vi "run.vi"(8 "error in (no error)":errorcluster, 11 "Protocol_TwoCreep in":refnum<class "Protocol_TwoCreep.lvclass">) -> (0 "error out":errorcluster, 3 "Protocol_TwoCreep out":refnum<class "Protocol_TwoCreep.lvclass">)   [LabVIEW 2011, in "Protocol_TwoCreep.lvclass"]
uses:
  Protocol_TwoCreep.lvclass
  protocol_Generic/Protocol_Generic.lvclass
  Protocol_TwoCreep.lvclass/Protocol_TwoCreep.ctl
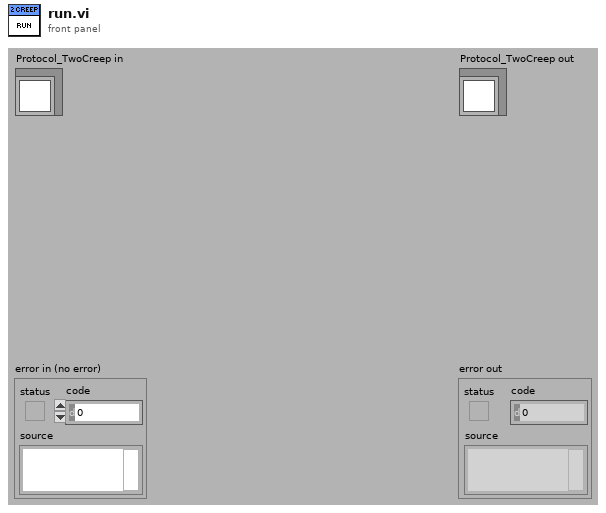
[diagram p1: front panel]
types:
  T1 = cluster{"Set Point":dbl, "Set Point Time":dbl, "Ramp Amplitude":dbl, "Ramp Rate":dbl}
  T2 = cluster{"Axis Information":cluster{"Device ID":i32, "Device Name":string, "Device Type":i32}[], "Axis Selector":i32[], "Control Modes out":u16[], "error out":errorcluster, "Channel Data":cluster{"Name":string, "Type":i32, "SI Full Scale":dbl, "Full Scale":dbl, "Units String":string, "Display Format":string, "Gauge Length":dbl}[][]}
  T3 = cluster{"Device ID":i32, "Device Name":string, "Device Type":i32}[]
  T4 = cluster{"Name":string, "Type":i32, "SI Full Scale":dbl, "Full Scale":dbl, "Units String":string, "Display Format":string, "Gauge Length":dbl}[][]
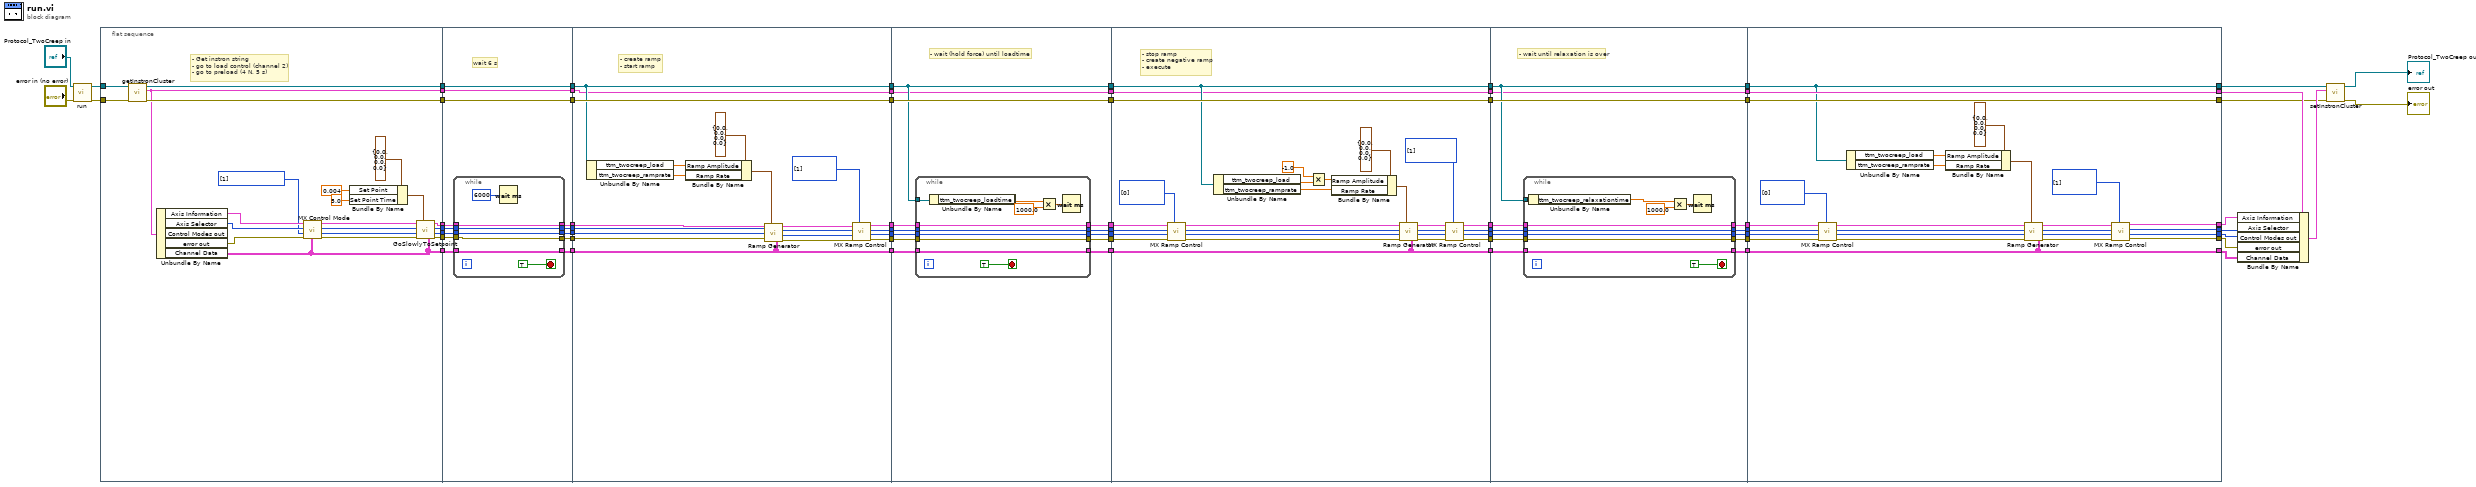
[diagram p0: block diagram]
diagram:
  n1 = call-parent "run.vi"("error in (no error)"="error in (no error)", "Protocol_Generic in"="Protocol_TwoCreep in") -> ("error out"=w60:errorcluster, "Protocol_Generic out"=w61:refnum<class "Protocol_TwoCreep.lvclass">)  [unwired: 8 in]
  n2 = flat-sequence {
    tunnel: w61 -> [w85]
    tunnel: w60 -> [w84]
    tunnel: [w64] -> w59
    tunnel: [w83] -> w58
    tunnel: [w70] -> w57
    tunnel: [w69] -> w56
    tunnel: [w68] -> w55
    tunnel: [w67] -> w54
    tunnel: [w66] -> w47
    tunnel: [w65] -> w17
    tunnel: w59 -> [w98]
    tunnel: w58 -> [w97]
    tunnel: w57 -> [w96]
    tunnel: w56 -> [w95]
    tunnel: w55 -> [w94]
    tunnel: w54 -> [w93]
    tunnel: [w98] -> w53
    tunnel: [w97] -> w52
    tunnel: [w92] -> w51
    tunnel: [w91] -> w50
    tunnel: [w90] -> w49
    tunnel: [w89] -> w48
    tunnel: w47 -> [w88]
    tunnel: [w87] -> w46
    tunnel: w17 -> [w86]
    tunnel: [w86] -> w16
    tunnel: w53 -> [w120]
    tunnel: w52 -> [w126]
    tunnel: w51 -> [w125]
    tunnel: w50 -> [w124]
    tunnel: w49 -> [w123]
    tunnel: w48 -> [w122]
    tunnel: w46 -> [w107]
    tunnel: [w120] -> w45
    tunnel: [w126] -> w44
    tunnel: [w111] -> w43
    tunnel: [w110] -> w42
    tunnel: [w109] -> w41
    tunnel: [w108] -> w40
    tunnel: [w107] -> w39
    tunnel: w16 -> [w106]
    tunnel: [w106] -> w15
    tunnel: w45 -> [w128]
    tunnel: w44 -> [w139]
    tunnel: w43 -> [w133]
    tunnel: w42 -> [w134]
    tunnel: w41 -> [w135]
    tunnel: w40 -> [w136]
    tunnel: w39 -> [w138]
    tunnel: [w128] -> w38
    tunnel: [w139] -> w37
    tunnel: [w137] -> w36
    tunnel: [w132] -> w35
    tunnel: [w131] -> w34
    tunnel: [w130] -> w33
    tunnel: [w129] -> w32
    tunnel: w15 -> [w127]
    tunnel: [w127] -> w13
    tunnel: w38 -> [w163]
    tunnel: w37 -> [w177]
    tunnel: w36 -> [w164]
    tunnel: w35 -> [w176]
    tunnel: w34 -> [w175]
    tunnel: w33 -> [w174]
    tunnel: w32 -> [w173]
    tunnel: [w163] -> w31
    tunnel: [w177] -> w30
    tunnel: [w164] -> w29
    tunnel: [w158] -> w28
    tunnel: [w156] -> w27
    tunnel: [w154] -> w26
    tunnel: [w152] -> w25
    tunnel: [w150] -> w14
    tunnel: w13 -> [w150]
    tunnel: w31 -> [w179]
    tunnel: w30 -> [w190]
    tunnel: w29 -> [w182]
    tunnel: w28 -> [w189]
    tunnel: w27 -> [w187]
    tunnel: w26 -> [w185]
    tunnel: w25 -> [w183]
    tunnel: [w179] -> w24
    tunnel: [w190] -> w23
    tunnel: [w181] -> w22
    tunnel: [w188] -> w21
    tunnel: [w186] -> w20
    tunnel: [w184] -> w19
    tunnel: [w180] -> w18
    tunnel: w14 -> [w178]
    tunnel: [w178] -> w12
    tunnel: [w204] -> w7
    tunnel: [w206] -> w8
    tunnel: [w208] -> w9
    tunnel: [w210] -> w10
    tunnel: [w203] -> w6
    tunnel: [w226] -> w1
    tunnel: [w201] -> w4
    tunnel: w24 -> [w201]
    tunnel: w23 -> [w226]
    tunnel: w22 -> [w203]
    tunnel: w21 -> [w216]
    tunnel: w20 -> [w215]
    tunnel: w19 -> [w214]
    tunnel: w18 -> [w213]
    tunnel: [w202] -> w11
    tunnel: w12 -> [w202]
    frame #0 {
      w79 = u16[] [1] items=["Channel 1", "Channel 2", "Channel 3", "Channel 4"] ("Control Modes")
      # "- Get instron string\n- go to load control (channel 2)\n- go to preload (4 N, 5 s)"
      n3 = call-dynamic "getInstronCluster.vi"("error in (no error)"=w84, "Protocol_Generic in"=w85) -> ("error out"=w83:errorcluster, "InstronCluster"=w65:T2, "Protocol_Generic out"=w64:refnum<class "Protocol_TwoCreep.lvclass">)  [unwired: 7 in]
      n4 = Unbundle By Name(w65) -> ("Axis Information"=w82:T3, "Axis Selector"=w81:i32[], "error out"=w80:errorcluster, "Channel Data"=w66:T4)  [unwired: 1 out]
      n5 = call "MX Control Mode.vi"("Channel Data"=w66, "error in (no error)"=w80, "Control Modes"=w79, "Axis Selector"=w81, "Axis Information"=w82) -> ("error out"=w75:errorcluster, "Control Modes out"=w76:u16[], "Axis Selector out"=w77:i32[], "Axis Information out"=w78:T3)  [unwired: 1 in]
      n6 = Bundle By Name(cluster=T1 {"Set Point"=0.0, "Set Point Time"=0.0, "Ramp Amplitude"=0.0, "Ramp Rate"=0.0} ("Input cluster"), "Set Point"=0.004, "Set Point Time"=5.0) -> (w74:T1)
      n7 = call "GoSlowlyToSetpoint.vi"("Channel Data"=w66, "Input cluster"=w74, "error in (no error)"=w75, "Channels"=w76, "Axis Selector"=w77, "Axis Information"=w78) -> ("Error Out"=w68:errorcluster, "Channels Out"=w67:u16[], "Axis Selector Out"=w69:i32[], "Axis Information Out"=w70:T3)  [unwired: 2 in]
    }
    frame #1 {
      # "wait 6 s"
      n8 = while {
        tunnel: w96 -> [w103]
        tunnel: w95 -> [w102]
        tunnel: w94 -> [w100]
        tunnel: w93 -> [w101]
        tunnel: [w103] -> w92
        tunnel: [w102] -> w91
        tunnel: [w101] -> w90
        tunnel: [w100] -> w89
        tunnel: w88 -> [w99]
        tunnel: [w99] -> w87
        stop <- TRUE stop-if-true
        n9 = Wait (ms)(milliseconds to wait=u32 6000) -> ()  [unwired: 1 out]
      }
    }
    frame #2 {
      w112 = u16[] [1] items=["Stop", "Start or continue", "Hold", "Continue", "Return ramp to set level at fixed rate", "Reserved", "Reserved", "Start Random without demand hold", "Start Random with demand hold", "Prepare Random Start without demand hold", "Prepare Random Start with demand hold", "Unslave", "Reserved", "Reserved", "Start Sample Data Playback or Resume", "Prepare for Start of Sample Data", "Reserved", "Reserved", "Resume Playback", "Start an electromechanical frame return"] ("Ramp Control")
      # "- create ramp\n- start ramp"
      n10 = Unbundle By Name(w120) -> ("ttm_twocreep_load"=w119:dbl, "ttm_twocreep_ramprate"=w118:dbl)
      n11 = Bundle By Name(cluster=T1 {"Set Point"=0.0, "Set Point Time"=0.0, "Ramp Amplitude"=0.0, "Ramp Rate"=0.0} ("Input cluster"), "Ramp Amplitude"=w119, "Ramp Rate"=w118) -> (w117:T1)
      n12 = call "Ramp Generator.vi"("Channel Data"=w107, "Input cluster"=w117, "error in (no error)"=w122, "Channels"=w123, "Axis Selector"=w124, "Axis Information"=w125) -> ("Error Out"=w113:errorcluster, "Channels Out"=w114:u16[], "Axis Selector Out"=w115:i32[], "Axis Information Out"=w116:T3)  [unwired: 2 in]
      n13 = call "MX Ramp Control.vi"("Ramp Control"=w112, "error in (no error)"=w113, "Channels In"=w114, "Axis Selector In"=w115, "Axis Information In"=w116) -> ("error out"=w108:errorcluster, "Channels Out"=w109:u16[], "Axis Selector Out"=w110:i32[], "Axis Information Out"=w111:T3)  [unwired: 2 in]
    }
    frame #3 {
      # "- wait (hold force) until loadtime"
      n14 = while {
        tunnel: w133 -> [w148]
        tunnel: w134 -> [w147]
        tunnel: w136 -> [w145]
        tunnel: w135 -> [w146]
        tunnel: [w148] -> w132
        tunnel: [w147] -> w131
        tunnel: [w146] -> w130
        tunnel: [w145] -> w129
        tunnel: w138 -> [w144]
        tunnel: [w144] -> w137
        tunnel: w128 -> [w143]
        stop <- TRUE stop-if-true
        n15 = Unbundle By Name(w143) -> ("ttm_twocreep_loadtime"=w142:dbl)
        n16 = Multiply(x=w142, y=1000.0) -> (x*y=w140:dbl)
        n17 = Wait (ms)(milliseconds to wait=w140) -> ()  [unwired: 1 out]
      }
    }
    frame #4 {
      w151 = u16[] [1] items=["Stop", "Start or continue", "Hold", "Continue", "Return ramp to set level at fixed rate", "Reserved", "Reserved", "Start Random without demand hold", "Start Random with demand hold", "Prepare Random Start without demand hold", "Prepare Random Start with demand hold", "Unslave", "Reserved", "Reserved", "Start Sample Data Playback or Resume", "Prepare for Start of Sample Data", "Reserved", "Reserved", "Resume Playback", "Start an electromechanical frame return"] ("Ramp Control")
      w172 = u16[] [0] items=["Stop", "Start or continue", "Hold", "Continue", "Return ramp to set level at fixed rate", "Reserved", "Reserved", "Start Random without demand hold", "Start Random with demand hold", "Prepare Random Start without demand hold", "Prepare Random Start with demand hold", "Unslave", "Reserved", "Reserved", "Start Sample Data Playback or Resume", "Prepare for Start of Sample Data", "Reserved", "Reserved", "Resume Playback", "Start an electromechanical frame return"] ("Ramp Control")
      # "- stop ramp\n- create negative ramp\n- execute"
      n18 = call "MX Ramp Control.vi"("Ramp Control"=w172, "error in (no error)"=w173, "Channels In"=w174, "Axis Selector In"=w175, "Axis Information In"=w176) -> ("error out"=w165:errorcluster, "Channels Out"=w166:u16[], "Axis Selector Out"=w167:i32[], "Axis Information Out"=w168:T3)  [unwired: 2 in]
      n19 = Unbundle By Name(w163) -> ("ttm_twocreep_load"=w162:dbl, "ttm_twocreep_ramprate"=w170:dbl)
      n20 = Multiply(x=-1.0, y=w162) -> (x*y=w161:dbl)
      n21 = Bundle By Name(cluster=T1 {"Set Point"=0.0, "Set Point Time"=0.0, "Ramp Amplitude"=0.0, "Ramp Rate"=0.0} ("Input cluster"), "Ramp Amplitude"=w161, "Ramp Rate"=w170) -> (w169:T1)
      n22 = call "Ramp Generator.vi"("Channel Data"=w164, "Input cluster"=w169, "error in (no error)"=w165, "Channels"=w166, "Axis Selector"=w167, "Axis Information"=w168) -> ("Error Out"=w153:errorcluster, "Channels Out"=w155:u16[], "Axis Selector Out"=w157:i32[], "Axis Information Out"=w159:T3)  [unwired: 2 in]
      n23 = call "MX Ramp Control.vi"("Ramp Control"=w151, "error in (no error)"=w153, "Channels In"=w155, "Axis Selector In"=w157, "Axis Information In"=w159) -> ("error out"=w152:errorcluster, "Channels Out"=w154:u16[], "Axis Selector Out"=w156:i32[], "Axis Information Out"=w158:T3)  [unwired: 2 in]
    }
    frame #5 {
      # "- wait until relaxation is over"
      n24 = while {
        tunnel: w189 -> [w199]
        tunnel: w187 -> [w198]
        tunnel: w183 -> [w191]
        tunnel: w185 -> [w197]
        tunnel: [w199] -> w188
        tunnel: [w198] -> w186
        tunnel: [w197] -> w184
        tunnel: [w191] -> w180
        tunnel: w182 -> [w196]
        tunnel: [w196] -> w181
        tunnel: w179 -> [w195]
        stop <- TRUE stop-if-true
        n25 = Unbundle By Name(w195) -> ("ttm_twocreep_relaxationtime"=w194:dbl)
        n26 = Multiply(x=w194, y=1000.0) -> (x*y=w192:dbl)
        n27 = Wait (ms)(milliseconds to wait=w192) -> ()  [unwired: 1 out]
      }
    }
    frame #6 {
      w212 = u16[] [0] items=["Stop", "Start or continue", "Hold", "Continue", "Return ramp to set level at fixed rate", "Reserved", "Reserved", "Start Random without demand hold", "Start Random with demand hold", "Prepare Random Start without demand hold", "Prepare Random Start with demand hold", "Unslave", "Reserved", "Reserved", "Start Sample Data Playback or Resume", "Prepare for Start of Sample Data", "Reserved", "Reserved", "Resume Playback", "Start an electromechanical frame return"] ("Ramp Control")
      w217 = u16[] [1] items=["Stop", "Start or continue", "Hold", "Continue", "Return ramp to set level at fixed rate", "Reserved", "Reserved", "Start Random without demand hold", "Start Random with demand hold", "Prepare Random Start without demand hold", "Prepare Random Start with demand hold", "Unslave", "Reserved", "Reserved", "Start Sample Data Playback or Resume", "Prepare for Start of Sample Data", "Reserved", "Reserved", "Resume Playback", "Start an electromechanical frame return"] ("Ramp Control")
      n28 = call "MX Ramp Control.vi"("Ramp Control"=w212, "error in (no error)"=w213, "Channels In"=w214, "Axis Selector In"=w215, "Axis Information In"=w216) -> ("error out"=w205:errorcluster, "Channels Out"=w207:u16[], "Axis Selector Out"=w209:i32[], "Axis Information Out"=w211:T3)  [unwired: 2 in]
      n29 = Unbundle By Name(w201) -> ("ttm_twocreep_load"=w224:dbl, "ttm_twocreep_ramprate"=w223:dbl)
      n30 = Bundle By Name(cluster=T1 {"Set Point"=0.0, "Set Point Time"=0.0, "Ramp Amplitude"=0.0, "Ramp Rate"=0.0} ("Input cluster"), "Ramp Amplitude"=w224, "Ramp Rate"=w223) -> (w222:T1)
      n31 = call "Ramp Generator.vi"("Channel Data"=w203, "Input cluster"=w222, "error in (no error)"=w205, "Channels"=w207, "Axis Selector"=w209, "Axis Information"=w211) -> ("Error Out"=w218:errorcluster, "Channels Out"=w219:u16[], "Axis Selector Out"=w220:i32[], "Axis Information Out"=w221:T3)  [unwired: 2 in]
      n32 = call "MX Ramp Control.vi"("Ramp Control"=w217, "error in (no error)"=w218, "Channels In"=w219, "Axis Selector In"=w220, "Axis Information In"=w221) -> ("error out"=w204:errorcluster, "Channels Out"=w206:u16[], "Axis Selector Out"=w208:i32[], "Axis Information Out"=w210:T3)  [unwired: 2 in]
    }
  }
  n33 = Bundle By Name(cluster=w11, "Axis Information"=w10, "Axis Selector"=w9, "Control Modes out"=w8, "error out"=w7, "Channel Data"=w6) -> (w2:T2)
  n34 = call-dynamic "setInstronCluster.vi"("error in (no error)"=w1, "InstronCluster"=w2, "Protocol_Generic in"=w4) -> ("error out"=→"error out":errorcluster, "Protocol_Generic out"=→"Protocol_TwoCreep out":refnum<class "Protocol_TwoCreep.lvclass">)  [unwired: 7 in]
